vi "piezo.vi"() -> ()   [LabVIEW 2017]
uses:
  C:/Users/Li Lab/Documents/LabVIEW Data/kinesis_test - 3/Thorlabs.MotionControl.Controls.dll
  Thorlabs.MotionControl.Controls.dll
  <vilib>/Utility/inputDevices.llb/closeJoystick.vi
  <vilib>/Utility/inputDevices.llb/joystickAcquire.vi
  C:/Users/Li Lab/Documents/LabVIEW Data/kinesis_test - 3/ThorLabs.MotionControl.KCube.DCServoCLI.dll
  ThorLabs.MotionControl.KCube.DCServoCLI.dll
  C:/Users/Li Lab/Documents/LabVIEW Data/kinesis_test - 3/Thorlabs.MotionControl.KCube.InertialMotorCLI.dll
  Thorlabs.MotionControl.KCube.InertialMotorCLI.dll
panel:
  out "x/y":dbl
  out "pov 1":i32
  in  "KCubeDCServoControl 2":refnum<k24>(container)
  in  "KCubeDCServoControl":refnum<k24>(container)
  out "direction info 2":T1
  out "axis info 2":T2
  in  "Tab Control 2":enum32{"Page 1", "Page 2"}(tab)
  in  "SerialNumber KDC101 2":string="27251775"
  in  "SerialNumber KDC101":string="27251750"
  in  "SerialNumber  of KIM101":string="97000019"
  in  "channel":i32(ring)=1 items=["Channel1"=1, "Channel2"=2, "Channel3"=3, "Channel4"=4]
  in  "Tab Control":enum32{"Page 1", "Page 2"}(tab)
  out "Numeric 4":dbl
  out "Numeric 2":dbl
  out "GetPosition":i32
  out "Numeric 3":dbl
  in  "stop 2":bool
  out "Numeric":dbl
  out "error out 4":errorcluster
  out "error out 2":errorcluster
  out "error out 3":errorcluster
  out "error out":errorcluster
  out "button info 2":T3
  in  "KCubeInertialMotorControl":refnum<k24>(container)
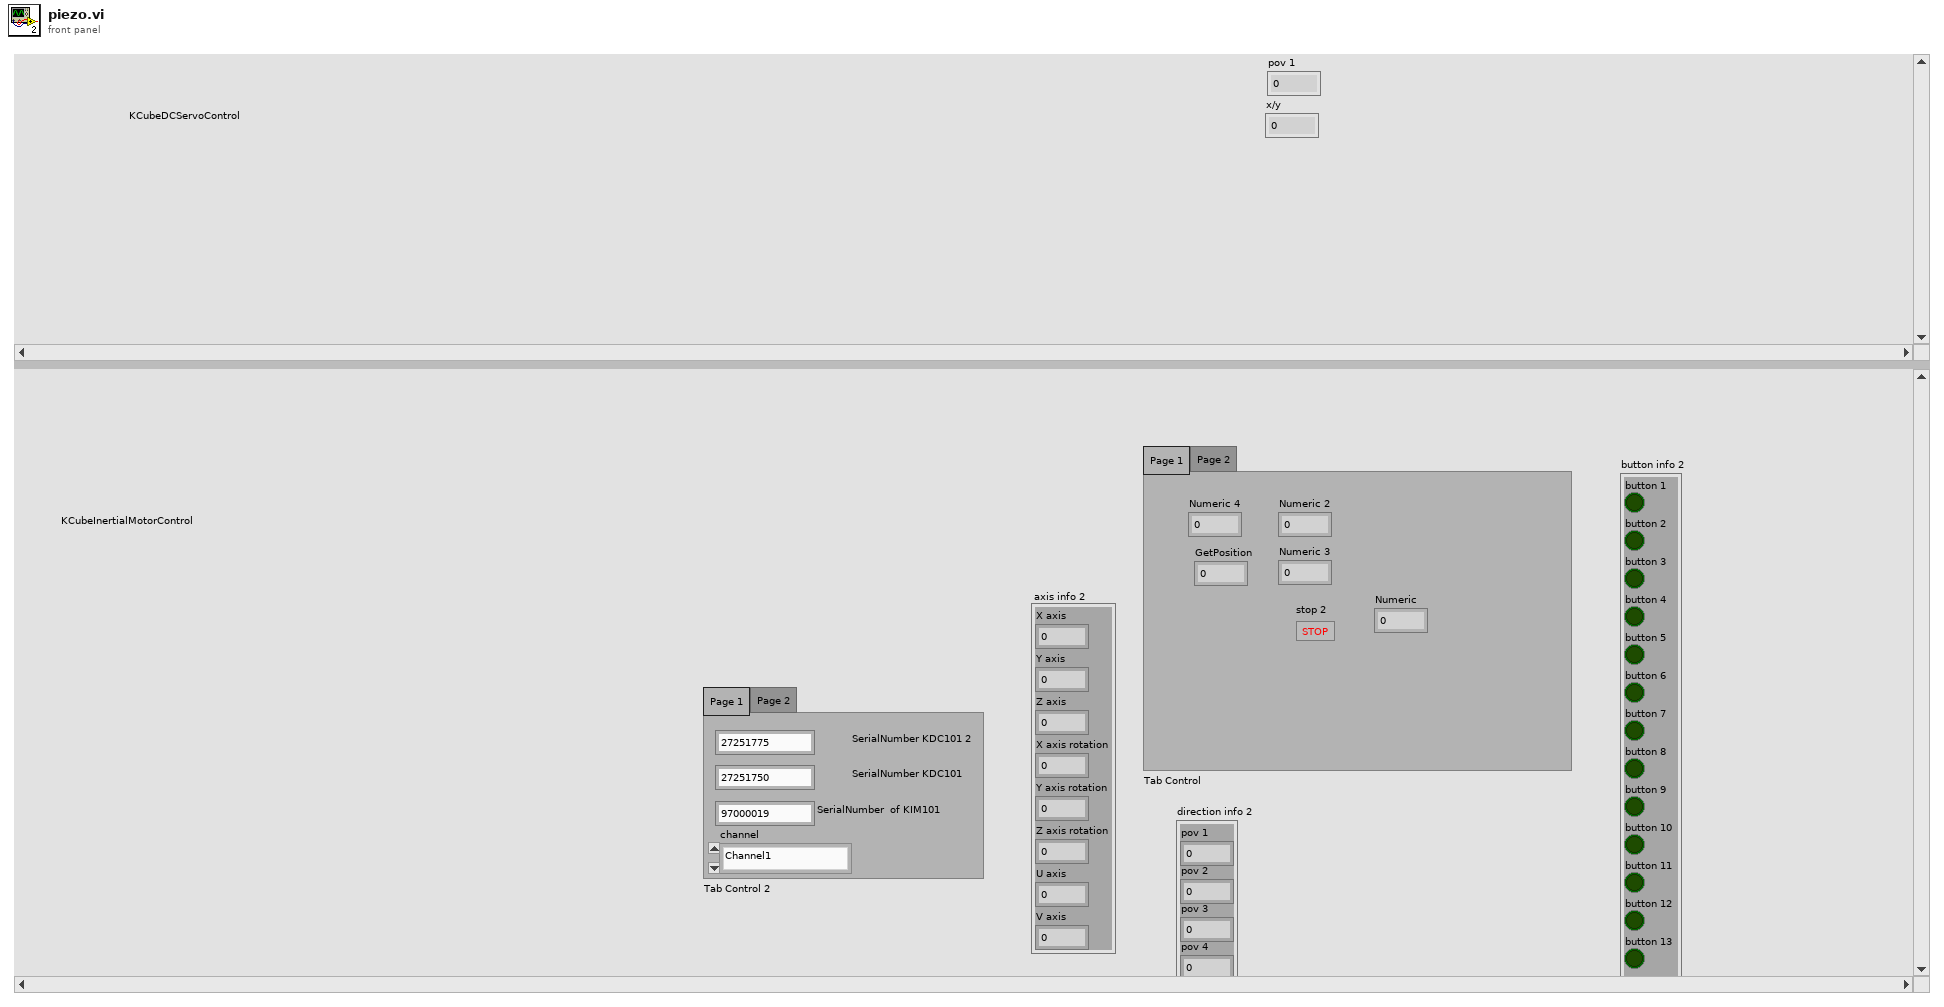
[diagram p1: front panel]
types:
  T1 = cluster{"pov 1":i32, "pov 2":i32, "pov 3":i32, "pov 4":i32}
  T2 = cluster{"X axis":i32, "Y axis":i32, "Z axis":i32, "X axis rotation":i32, "Y axis rotation":i32, "Z axis rotation":i32, "U axis":i32, "V axis":i32}
  T3 = cluster{"button 1":bool, "button 2":bool, "button 3":bool, "button 4":bool, "button 5":bool, "button 6":bool, "button 7":bool, "button 8":bool, "button 9":bool, "button 10":bool, "button 11":bool, "button 12":bool, "button 13":bool, "button 14":bool, "button 15":bool, "button 16":bool, "button 17":bool, "button 18":bool, "button 19":bool, "button 20":bool, "button 21":bool, "button 22":bool, "button 23":bool, "button 24":bool, "button 25":bool, "button 26":bool, "button 27":bool, "button 28":bool, "button 29":bool, "button 30":bool, "button 31":bool, "button 32":bool}
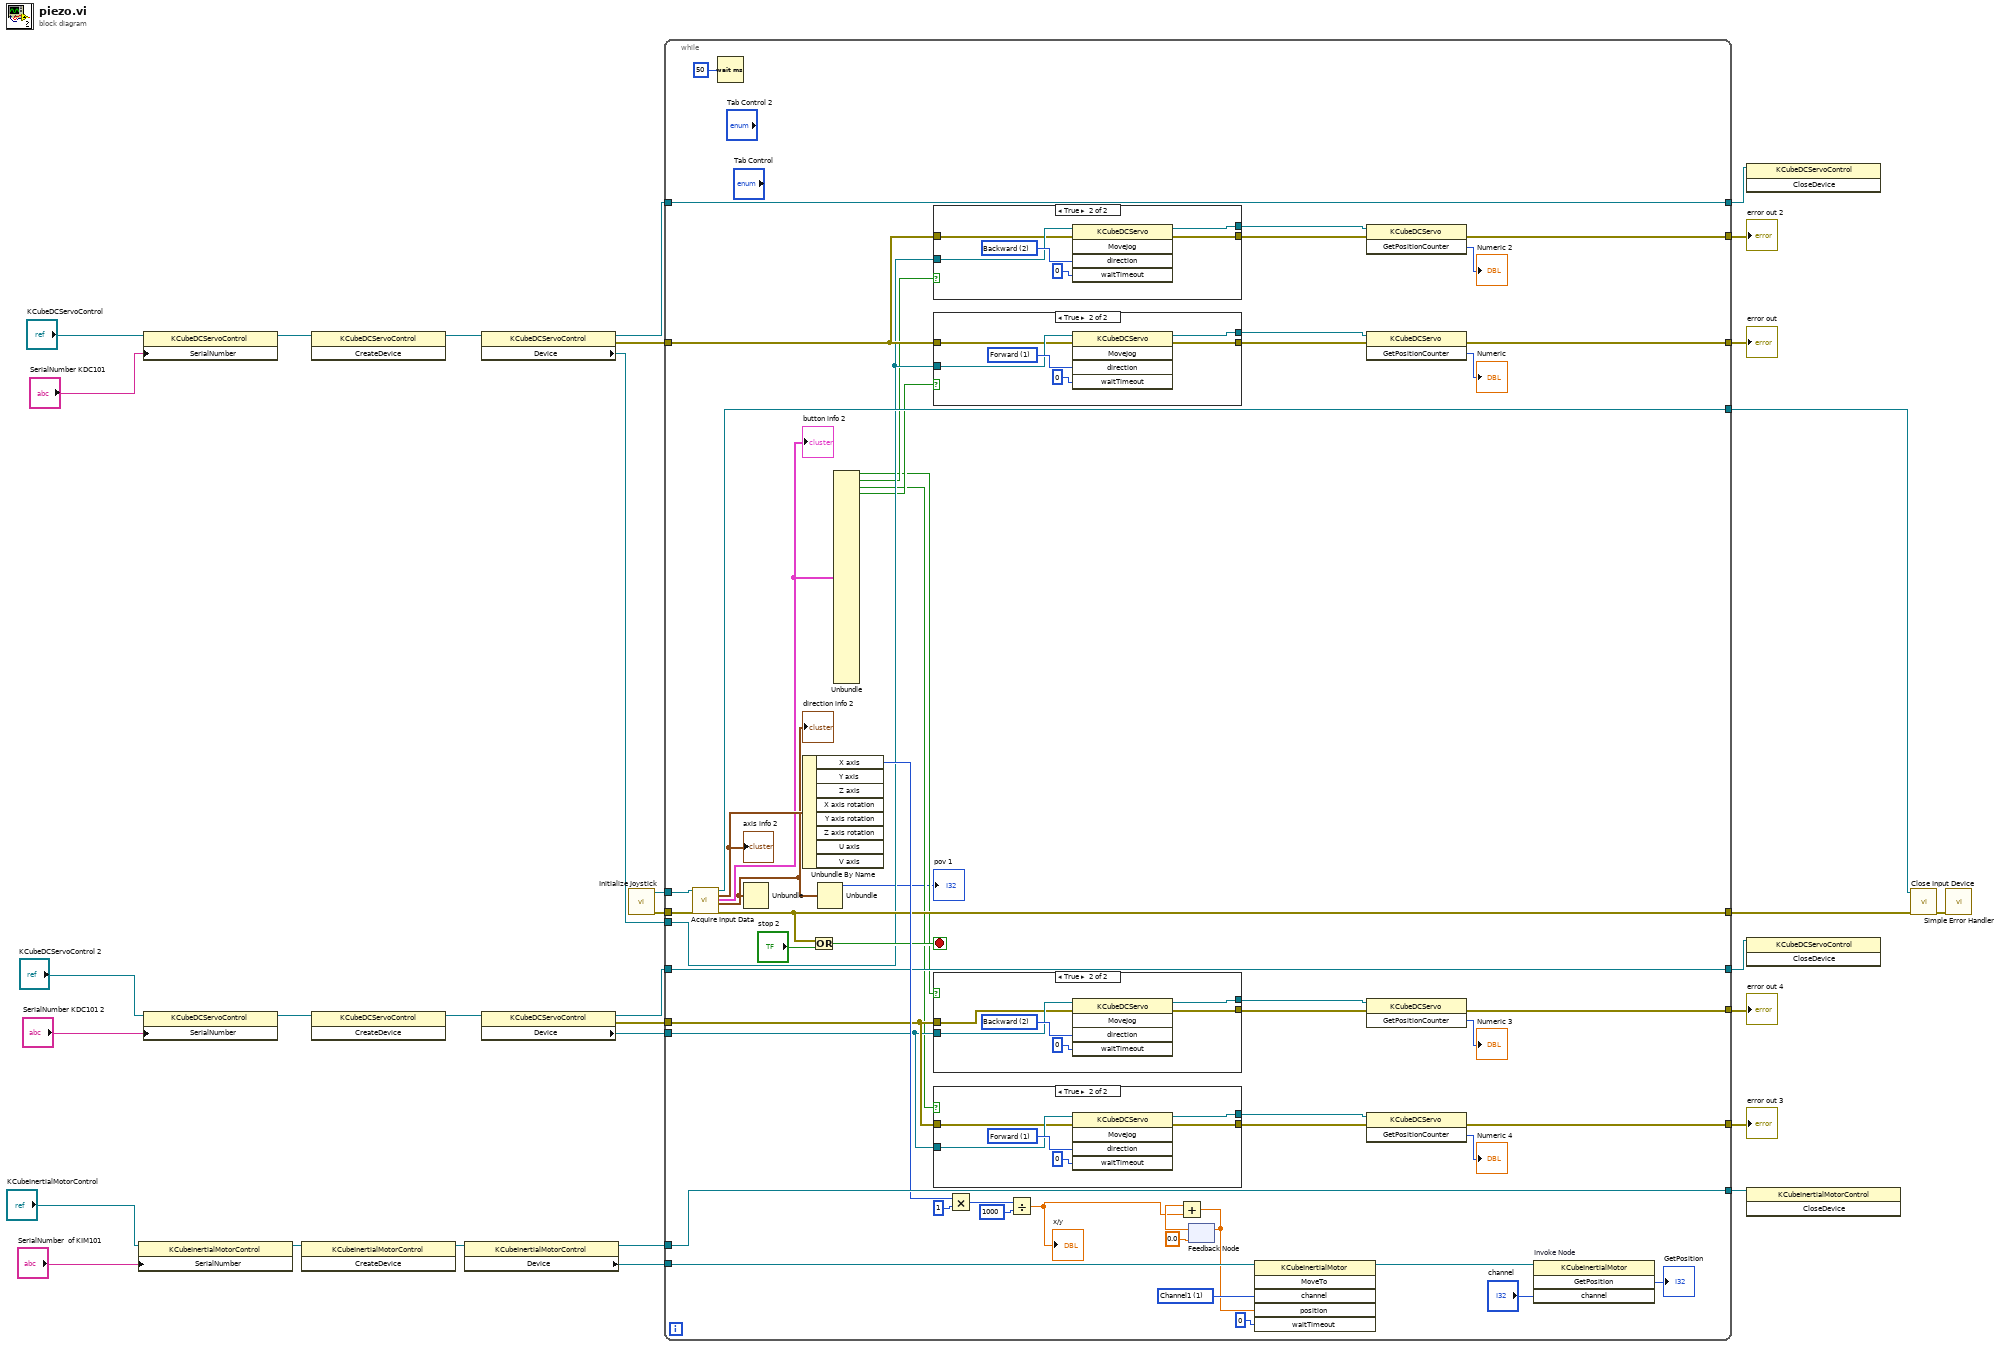
[diagram p0: block diagram]
diagram:
  n1 = property class="KCubeInertialMotorControl"(reference="KCubeInertialMotorControl", "SerialNumber"="SerialNumber  of KIM101") -> (reference out=w30:refnum<k24>)  [unwired: 1 in, 1 out]
  n2 = property class="KCubeDCServoControl"(reference="KCubeDCServoControl", "SerialNumber"="SerialNumber KDC101") -> (reference out=w25:refnum<k24>)  [unwired: 1 in, 1 out]
  n3 = property class="KCubeDCServoControl"(reference="KCubeDCServoControl 2", "SerialNumber"="SerialNumber KDC101 2") -> (reference out=w20:refnum<k24>)  [unwired: 1 in, 1 out]
  n4 = invoke class="KCubeInertialMotorControl" method="CreateDevice"(reference=w30) -> (reference out=w29:refnum<k24>)  [unwired: 2 in, 2 out]
  n5 = invoke class="KCubeDCServoControl" method="CreateDevice"(reference=w25) -> (reference out=w26:refnum<k24>)  [unwired: 2 in, 2 out]
  n6 = invoke class="KCubeDCServoControl" method="CreateDevice"(reference=w20) -> (reference out=w19:refnum<k24>)  [unwired: 2 in, 2 out]
  n7 = property class="KCubeInertialMotorControl"(reference=w29) -> (reference out=w28:refnum<k24>, "Device"=w18:refnum<k24>)  [unwired: 1 in, 1 out]
  n8 = property class="KCubeDCServoControl"(reference=w26) -> (reference out=w12:refnum<k24>, error out=w8:errorcluster, "Device"=w10:refnum<k24>)  [unwired: 1 in]
  n9 = property class="KCubeDCServoControl"(reference=w19) -> (reference out=w6:refnum<k24>, error out=w4:errorcluster, "Device"=w3:refnum<k24>)  [unwired: 1 in]
  n10 = call <vilib>:"Initialize Joystick.vi"() -> ("error out"=w13:errorcluster, "device ID"=w14:refnum<k1>)  [unwired: 10 in]
  n11 = while {
    tunnel: w28 -> [w84]
    tunnel: [w84] -> w27
    tunnel: w18 -> [w41]
    tunnel: [w72] -> w16
    tunnel: [w73] -> w15
    tunnel: w14 -> [w76]
    tunnel: w13 -> [w75]
    tunnel: w12 -> [w71]
    tunnel: [w71] -> w11
    tunnel: w10 -> [w61]
    tunnel: [w69] -> w9
    tunnel: w8 -> [w62]
    tunnel: [w60] -> w7
    tunnel: [w53] -> w5
    tunnel: w6 -> [w53]
    tunnel: w4 -> [w52]
    tunnel: w3 -> [w51]
    tunnel: [w50] -> w2
    tunnel: [w49] -> w1
    stop <- w74 stop-if-true
    w39 = 1 items=["Channel1"=1, "Channel2"=2, "Channel3"=3, "Channel4"=4] ("channel")
    n12 = call-poly <vilib>:"Acquire Input Data.vi"("device ID"=w76, "error in (no error)"=w75) -> ("device ID"=w73:refnum<k1>, "axis info"=w78:T2, "button info"=w68:T3, "direction info"=w44:T1, "error out"=w72:errorcluster)  [unwired: 13 in]
    "axis info 2" <- w78
    "direction info 2" <- w44
    "button info 2" <- w68
    n13 = Wait (ms)(milliseconds to wait=u32 50) -> ()  [unwired: 1 out]
    n14 = Unbundle(w44) -> ()  [unwired: 4 out]
    n15 = Unbundle By Name(w78) -> ("X axis"=w79:i32)  [unwired: 7 out]
    n16 = Or(x=w72, y="stop 2") -> (x .or. y?=w74:bool)
    n17 = Unbundle(w44) -> ("pov 1"=→"pov 1":i32)  [unwired: 3 out]
    n18 = Unbundle(w68) -> ("button 1"=w45:bool, "button 2"=w47:bool, "button 3"=w46:bool, "button 4"=w48:bool)  [unwired: 28 out]
    n19 = case shown="True" w47 {
      tunnel: [w102 w108] -> w64
      tunnel: w61 -> [w102 w105]
      tunnel: [w101 w104] -> w65
      tunnel: w62 -> [w101 w103]
      frame False {
      }
      frame True {
        w107 = 2 items=["Forward"=1, "Backward"=2] ("direction")
        n20 = invoke class="KCubeDCServo" method="MoveJog"(reference=w105, error in=w103, "direction"=w107, "waitTimeout"=0) -> (reference out=w108:refnum<k24>, error out=w104:errorcluster)  [unwired: 1 in, 3 out]
      }
    }
    n21 = case shown="True" w48 {
      tunnel: [w110 w116] -> w67
      tunnel: w61 -> [w110 w113]
      tunnel: [w109 w112] -> w66
      tunnel: w62 -> [w109 w111]
      frame False {
      }
      frame True {
        w115 = 1 items=["Forward"=1, "Backward"=2] ("direction")
        n22 = invoke class="KCubeDCServo" method="MoveJog"(reference=w113, error in=w111, "direction"=w115, "waitTimeout"=0) -> (reference out=w116:refnum<k24>, error out=w112:errorcluster)  [unwired: 1 in, 3 out]
      }
    }
    n23 = case shown="True" w45 {
      tunnel: [w86 w92] -> w58
      tunnel: w51 -> [w86 w89]
      tunnel: [w85 w88] -> w57
      tunnel: w52 -> [w85 w87]
      frame False {
      }
      frame True {
        w91 = 2 items=["Forward"=1, "Backward"=2] ("direction")
        n24 = invoke class="KCubeDCServo" method="MoveJog"(reference=w89, error in=w87, "direction"=w91, "waitTimeout"=0) -> (reference out=w92:refnum<k24>, error out=w88:errorcluster)  [unwired: 1 in, 3 out]
      }
    }
    n25 = case shown="True" w46 {
      tunnel: [w94 w100] -> w55
      tunnel: w51 -> [w94 w97]
      tunnel: [w93 w96] -> w56
      tunnel: w52 -> [w93 w95]
      frame False {
      }
      frame True {
        w99 = 1 items=["Forward"=1, "Backward"=2] ("direction")
        n26 = invoke class="KCubeDCServo" method="MoveJog"(reference=w97, error in=w95, "direction"=w99, "waitTimeout"=0) -> (reference out=w100:refnum<k24>, error out=w96:errorcluster)  [unwired: 1 in, 3 out]
      }
    }
    n27 = Multiply(x=w79, y=1) -> (x*y=w80:i32)
    n28 = Divide(x=w80, y=1000) -> (x/y=w35:dbl)
    "x/y" <- w35
    n29 = feedback #1(0.0) -> (w36:dbl)
    n30 = Add(x=w36, y=w35) -> (x+y=w34:dbl)
    n31 = feedback-in #1(w34) -> ()
    n32 = invoke class="KCubeInertialMotor" method="MoveTo"(reference=w41, "channel"=w39, "position"=w34, "waitTimeout"=0) -> (reference out=w40:refnum<k24>)  [unwired: 2 in, 5 out]
    n33 = invoke class="KCubeDCServo" method="GetPositionCounter"(reference=w64, error in=w65) -> (error out=w60:errorcluster, "GetPositionCounter"=→"Numeric 2":i32)  [unwired: 1 in, 1 out]
    n34 = invoke class="KCubeDCServo" method="GetPositionCounter"(reference=w67, error in=w66) -> (error out=w69:errorcluster, "GetPositionCounter"=→"Numeric":i32)  [unwired: 1 in, 1 out]
    n35 = invoke class="KCubeDCServo" method="GetPositionCounter"(reference=w58, error in=w57) -> (error out=w49:errorcluster, "GetPositionCounter"=→"Numeric 3":i32)  [unwired: 1 in, 1 out]
    n36 = invoke class="KCubeDCServo" method="GetPositionCounter"(reference=w55, error in=w56) -> (error out=w50:errorcluster, "GetPositionCounter"=→"Numeric 4":i32)  [unwired: 1 in, 1 out]
    n37 = invoke on="Invoke Node" class="KCubeInertialMotor" method="GetPosition"(reference=w40, "channel"="channel") -> ("GetPosition"=→"GetPosition":i32)  [unwired: 2 in, 3 out]
  }
  "error out" <- w9
  "error out 2" <- w7
  "error out 3" <- w2
  "error out 4" <- w1
  n38 = invoke class="KCubeDCServoControl" method="CloseDevice"(reference=w11) -> ()  [unwired: 2 in, 3 out]
  n39 = invoke class="KCubeDCServoControl" method="CloseDevice"(reference=w5) -> ()  [unwired: 2 in, 3 out]
  n40 = invoke class="KCubeInertialMotorControl" method="CloseDevice"(reference=w27) -> ()  [unwired: 2 in, 3 out]
  n41 = call-poly <vilib>:"Close Input Device.vi"("error in (no error)"=w16, "device ID"=w15) -> ("error out"=w17:errorcluster)  [unwired: 8 in]
  n42 = call <vilib>:"Simple Error Handler.vi"("error in (no error)"=w17) -> ()  [unwired: 4 in, 5 out]
